vi "File Handling Module.vi"(8 "error in (no error)":errorcluster, 11 "Queue in":refnum<queue>) -> (0 "error out":errorcluster)   [LabVIEW 2020]
uses:
  Libraries/Message Queue/Message Cluster.ctl
  <vilib>/Utility/error.llb/Error Cluster From Error Code.vi
  <vilib>/ErrorRing/Error Ring.xnode
  Libraries/Message Queue/Message Queue.lvlib
  Controls/File Handling Data.ctl
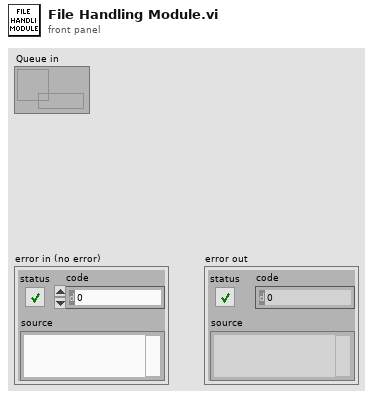
[diagram p1: front panel]
types:
  T1 = typedef "File Handling Data.ctl" = cluster{"Boolean <Replace Me>":bool, "String <Replace Me>":string, "Numeric <Replace Me>":dbl}
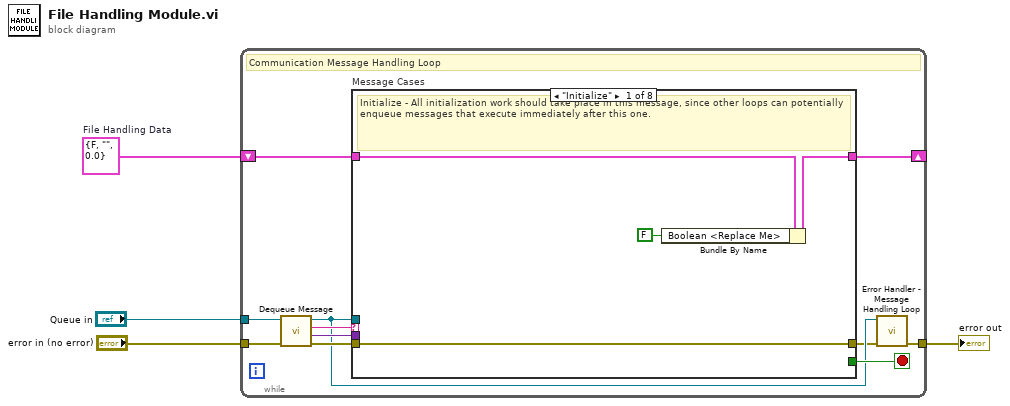
[diagram p0: block diagram]
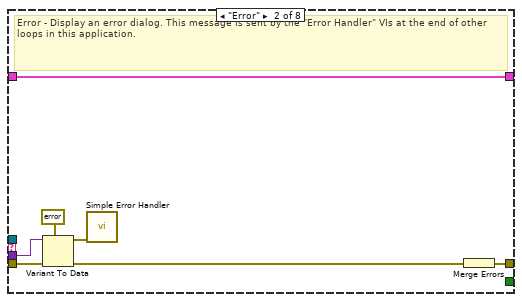
[diagram p2: hidden frame]
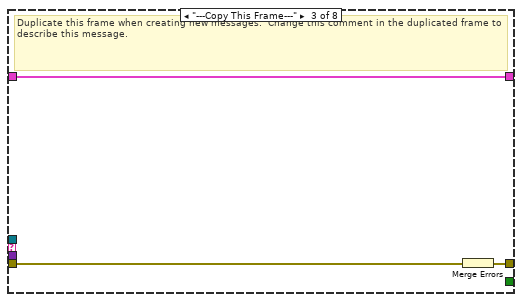
[diagram p3: hidden frame]
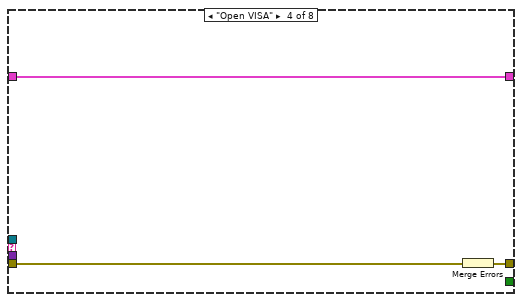
[diagram p4: hidden frame]
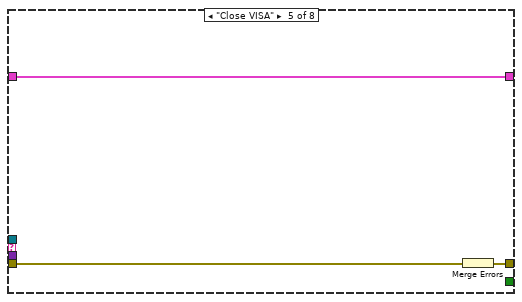
[diagram p5: hidden frame]
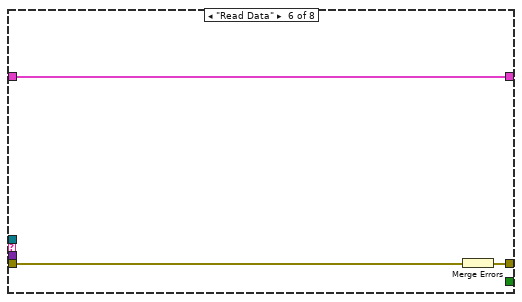
[diagram p6: hidden frame]
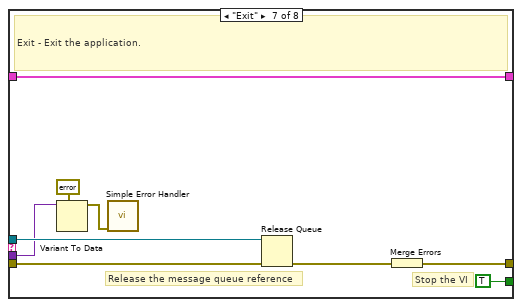
[diagram p7: hidden frame]
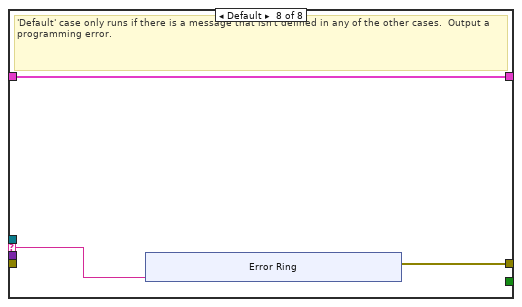
[diagram p8: hidden frame]
diagram:
  w1 = T1 {"Boolean <Replace Me>"=FALSE, "String <Replace Me>"="", "Numeric <Replace Me>"=0.0}  # File Handling Data
  n1 = while {
    tunnel: "Queue in" -> [w8]
    shift-right: [w14] -> _
    shift-left: w1 -> [w15]
    tunnel: "error in (no error)" -> [w12]
    tunnel: [w6] -> w4
    stop <- w13 stop-if-true
    # "Communication Message Handling Loop"
    n2 = call "Dequeue Message.vi"("error in (no error)"=w12, "Message Queue"=w8) -> ("error out"=w11:errorcluster, "Message Data"=w9:variant, "Message"=w10:string, "dup Message Queue"=w7:refnum<queue>)  [unwired: 6 in]
    n3 = case "Message Cases" shown="\"Initialize\"" w10 {
      selector: w10 -> [_ _ _ _ _ _ _ w48]
      tunnel: w7 -> [_ _ _ _ _ _ w47 _]
      tunnel: w11 -> [w19 w26 w29 w32 w35 w38 w43 _]
      tunnel: [w19 w20 w27 w30 w33 w36 w44 w49] -> w5
      tunnel: w15 -> [w18 w25 w28 w31 w34 w37 w39 w50]
      tunnel: [w17 w25 w28 w31 w34 w37 w39 w50] -> w14
      tunnel: [_ _ _ _ _ _ TRUE _] -> w13
      tunnel: w9 -> [_ w24 _ _ _ _ w40 _]
      frame "Initialize" {
        # "Initialize - All initialization work should take place in this message, since other loops can potentially enqueue messages that execute immediately after this one."
        n4 = Bundle By Name(cluster=w18, "Boolean <Replace Me>"=FALSE) -> (w17:T1)
      }
      frame "Error" {
        # "Error - Display an error dialog. This message is sent by the \"Error Handler\" VIs at the end of other loops in this application."
        n5 = Variant To Data(error in=w26, type=errorcluster {"status"=FALSE, "code"=0, "source"=""} ("error constant"), Variant=w24) -> (data=w22:errorcluster, error out=w21:errorcluster)
        n6 = call <vilib>:"Simple Error Handler.vi"("error in (no error)"=w22) -> ()  [unwired: 4 in, 5 out]
        n7 = Merge Errors(w21) -> (w20:errorcluster)
      }
      frame "---Copy This Frame---" {
        # "Duplicate this frame when creating new messages.  Change this comment in the duplicated frame to describe this message."
        n8 = Merge Errors(w29) -> (w27:errorcluster)
      }
      frame "Open VISA" {
        n9 = Merge Errors(w32) -> (w30:errorcluster)
      }
      frame "Close VISA" {
        n10 = Merge Errors(w35) -> (w33:errorcluster)
      }
      frame "Read Data" {
        n11 = Merge Errors(w38) -> (w36:errorcluster)
      }
      frame "Exit" {
        # "Stop the VI"
        # "Release the message queue reference"
        # "Exit - Exit the application."
        n12 = Variant To Data(type=errorcluster {"status"=FALSE, "code"=0, "source"=""} ("error constant"), Variant=w40) -> (data=w41:errorcluster)  [unwired: 1 in, 1 out]
        n13 = call <vilib>:"Simple Error Handler.vi"("error in (no error)"=w41) -> ()  [unwired: 4 in, 5 out]
        n14 = Release Queue(queue=w47, error in (no error)=w43) -> (error out=w45:errorcluster)  [unwired: 1 in, 2 out]
        n15 = Merge Errors(w45) -> (w44:errorcluster)
      }
      frame Default {
        # "'Default' case only runs if there is a message that isn't defined in any of the other cases.  Output a programming error."
        n16 = xnode "Error Ring"("parameter 0"=w48) -> ("error out"=w49:errorcluster)
      }
    }
    n17 = call "Error Handler - Message Handling Loop.vi"("error in (no error)"=w5, "Message Queue"=w7) -> ("dup error in"=w6:errorcluster)  [unwired: 8 in, 1 out]
  }
  "error out" <- w4
